vi "setup_configuration.vi"(8 "error in (no error)":errorcluster, 11 "SIMU_MIRROR in":refnum<class "SIMU_MIRROR.lvclass">) -> (0 "error out":errorcluster, 3 "SIMU_MIRROR out":refnum<class "SIMU_MIRROR.lvclass">)   [LabVIEW 2020, in "SIMU_MIRROR.lvclass"]
uses:
  SIMU_MIRROR.lvclass
  mirror.lvclass
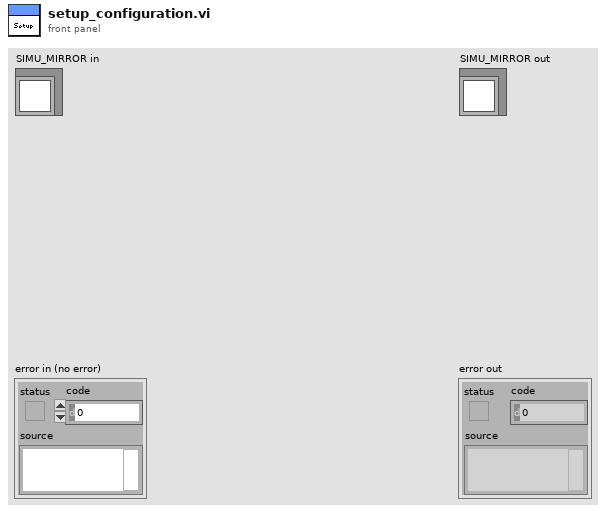
[diagram p1: front panel]
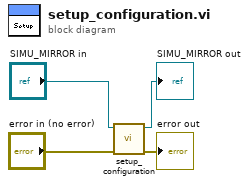
[diagram p0: block diagram]
diagram:
  n1 = call-parent "setup_configuration.vi"("error in (no error)"="error in (no error)", "mirror in"="SIMU_MIRROR in") -> ("error out"=→"error out":errorcluster, "mirror out"=→"SIMU_MIRROR out":refnum<class "SIMU_MIRROR.lvclass">)  [unwired: 8 in]
